vi "String Get Lines.vi"(11 "string":string) -> (1 "number of lines":i32, 3 "lines":string[](array[string]))   [LabVIEW 2014, in "C Header Generator.lvlib"]
uses:
  C Header Generator.lvlib
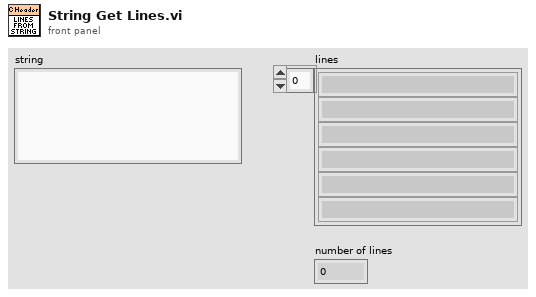
[diagram p1: front panel]
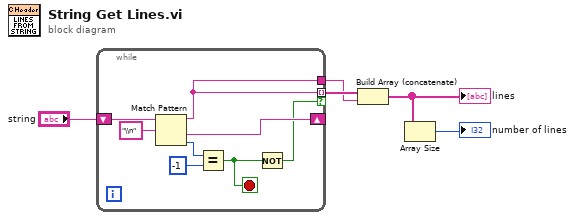
[diagram p0: block diagram]
diagram:
  n1 = while {
    shift-right: [w11] -> _
    shift-left: "string" -> [w12]
    tunnel: [w6] -> w4 mode=indexing if=w7
    tunnel: [w6] -> w3
    stop <- w8 stop-if-true
    n2 = Match Pattern(string=w12, regular expression="\\n") -> (before substring=w6:string, after substring=w11:string, offset past match=w10:i32)  [unwired: 1 in, 1 out]
    n3 = Equal?(x=w10, y=-1) -> (x = y?=w8:bool)
    n4 = Not(x=w8) -> (.not. x?=w7:bool)
  }
  n5 = Build Array (concatenate)(w4, w3) -> (w2:string[])
  "lines" <- w2
  n6 = Array Size(array=w2) -> (size(s)=→"number of lines":i32)
